vi "2D Array.vi"() -> (0 "error out":errorcluster)   [LabVIEW 2017, in "Assertion.Tests.lvlib" / "Assert Count.lvlib"]
uses:
  Assert Count.lvlib
  Assertion/Assertion.lvlib
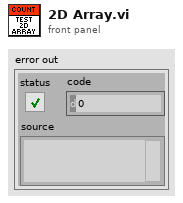
[diagram p1: front panel]
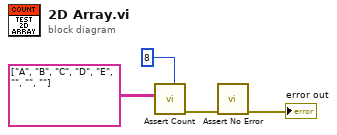
[diagram p0: block diagram]
diagram:
  n1 = call "Assert Count.vi"("Expected"=8, "Haystack"=string[][] [["A", "B", "C", "D"], ["E", "", "", ""]]) -> ("error out"=w2:errorcluster)  [unwired: 9 in]
  n2 = call "Assert No Error.vi"("error in (no error)"=w2) -> ("error out"=→"error out":errorcluster)  [unwired: 10 in]
